vi "Test Process Reentrancy.vi"(8 "error in (no error)":errorcluster, 11 "Process Test in":refnum<class "Process Test.lvclass">) -> (0 "error out":errorcluster, 3 "Process Test out":refnum<class "Process Test.lvclass">)   [LabVIEW 2020, in "Process Test.lvclass"]
uses:
  Process Test.lvclass
  C:/Users/anton/Documents/GitHub/Triarc-Framework/source/Framework Test/Base Class Test/Base Class Test.lvclass
  C:/Program Files (x86)/National Instruments/LabVIEW 2020/vi.lib/Asteme/LUnit/Test Case.lvclass
  Base Class Test/Base Class Test.lvclass/Base Class Test.ctl
  <vilib>/Asteme/LUnit/Test Case.lvclass/Test Case.ctl
  <vilib>/Asteme/LUnit/LUnit Assertion Result.lvclass/LUnit Assertion Result.ctl
  <vilib>/Asteme/LUnit/Palette/Fail.vi
  <vilib>/Asteme/LUnit/Palette/Pass.vi
  <vilib>/Asteme/LUnit/Set Assertion Type.vi
  <vilib>/Asteme/LUnit/Add test result.vi
  <vilib>/Asteme/LUnit/LUnit Write Passed.vi
  <vilib>/Asteme/LUnit/LUnit Get Test Case.vi
  <vilib>/Asteme/LUnit/LUnit Write Message.vi
  <vilib>/Asteme/LUnit/LUnit Write Description.vi
  <vilib>/Asteme/LUnit/LUnit Write Assertion Type.vi
  <vilib>/Asteme/LUnit/Read Test Case Name.vi
  <vilib>/Asteme/LUnit/Assertion Result/LUnit Get Test Name.vi
  Framework/Base/Base.lvclass
  <vilib>/Asteme/LUnit/LUnit Assertion Result.lvclass
  <vilib>/Asteme/LUnit/Test Case.lvclass
  Base Class Test/Base Class Test.lvclass
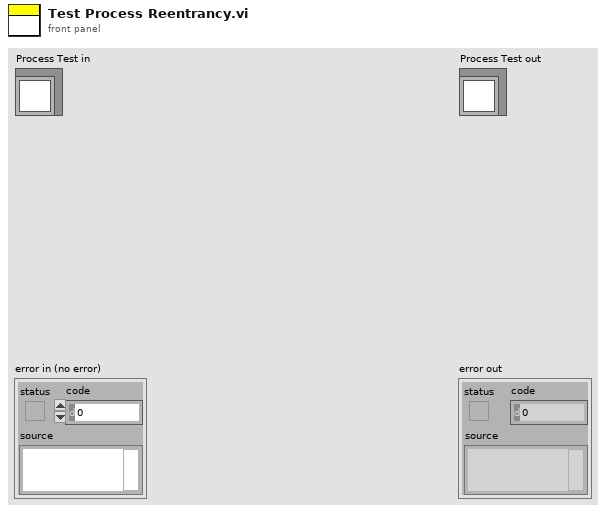
[diagram p1: front panel]
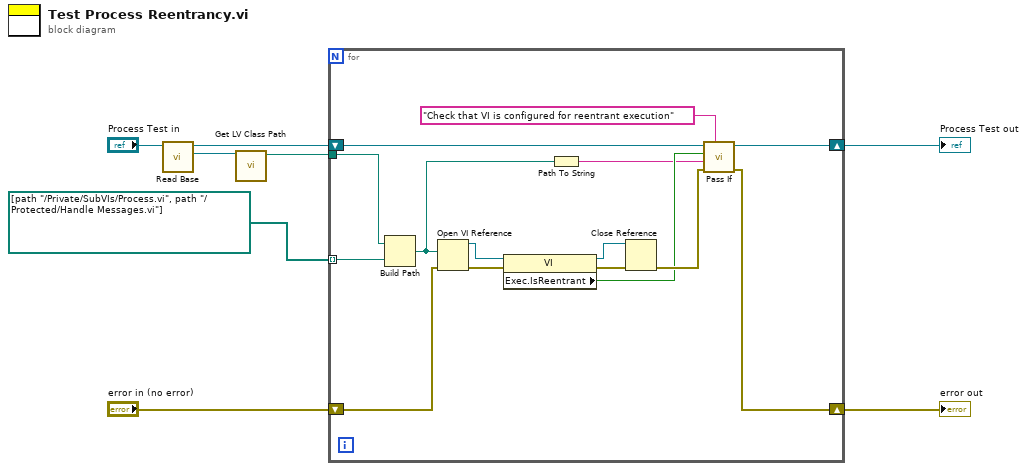
[diagram p0: block diagram]
diagram:
  n1 = call "Read Base.vi"("Base Class Test In"="Process Test in") -> ("Base.lvclass"=w3:refnum<class "Base.lvclass">, "Base Class Test Out"=w4:refnum<class "Process Test.lvclass">)  [unwired: 8 in, 1 out]
  n2 = call <vilib>:"Get LV Class Path.vi"("object"=w3) -> ("class path"=w2:path)  [unwired: 9 in, 1 out]
  n3 = for {
    tunnel: w2 -> [w12]
    shift-right: [w18] -> w6
    shift-left: "error in (no error)" -> [w16]
    shift-right: [w21] -> w7
    shift-left: w4 -> [w13]
    tunnel: path[] [path "../Private/SubVIs/Process.vi", path "../Protected/Handle Messages.vi"] -> [w11] mode=indexing
    n4 = Build Path(base path=w12, name or relative path=w11) -> (appended path=w10:path)
    n5 = Open VI Reference(vi path=w10, error in (no error)=w16) -> (vi reference=w15:refnum<vi>, error out=w17:errorcluster)  [unwired: 4 in]
    n6 = property class="VI"(reference=w15, error in=w17) -> (reference out=w22:refnum<vi>, error out=w23:errorcluster, "Exec.IsReentrant"=w19:bool)
    n7 = Path To String(path=w10) -> (string=w9:string)
    n8 = Close Reference(reference=w22, error in (no error)=w23) -> (error out=w20:errorcluster)
    n9 = call <vilib>:"Pass If.vi"("Description"="Check that VI is configured for reentrant execution", "error in (no error)"=w20, "Message"=w9, "Pass?"=w19, "Test Case In"=w13) -> ("error out"=w18:errorcluster, "Test Case Out"=w21:refnum<class "Process Test.lvclass">)  [unwired: 5 in]
  }
  "error out" <- w6
  "Process Test out" <- w7
